vi "Read_MessageHandler_MessageNb.vi"(8 "error in (no error)":errorcluster, 11 "MessageHandler in":refnum<class "MessageHandler.lvclass">) -> (0 "error out":errorcluster, 2 "Message number":u32, 3 "MessageHandler out":refnum<class "MessageHandler.lvclass">)   [LabVIEW 2013, in "MessageHandler.lvclass"]
uses:
  MessageHandler.lvclass
  MessageHandler.lvclass/MessageHandler.ctl
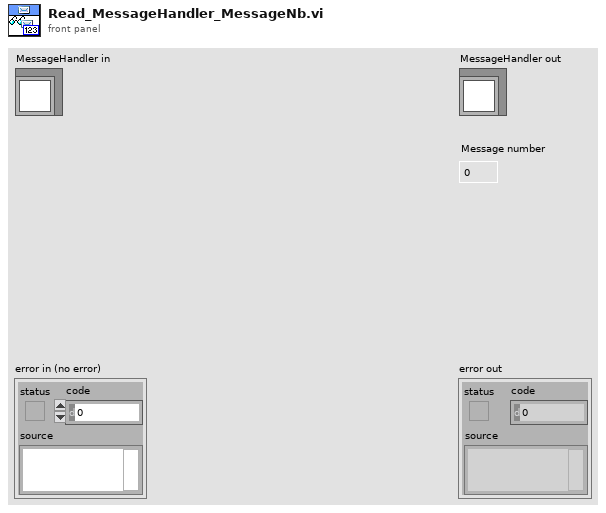
[diagram p1: front panel]
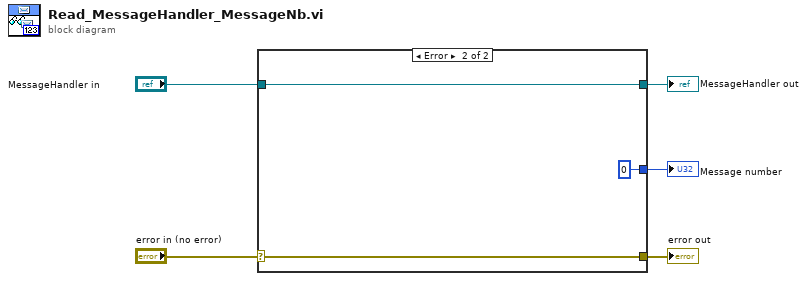
[diagram p0: block diagram]
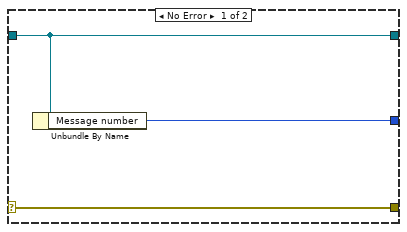
[diagram p2: hidden frame]
diagram:
  n1 = case shown="Error" "error in (no error)" {
    selector: "error in (no error)" -> [w8 w10]
    tunnel: [w8 w10] -> w4
    tunnel: [w7 w11] -> w2
    tunnel: "MessageHandler in" -> [w7 w11]
    tunnel: [w6 u32 0 ("Message number")] -> w1
    frame No Error {
      n2 = Unbundle By Name(w7) -> ("Message number"=w6:u32)
    }
    frame Error {
    }
  }
  "error out" <- w4
  "MessageHandler out" <- w2
  "Message number" <- w1
